vi "network stream read bulk.vi"(0 "endpoint in":refnum<k21>, 1 "Data num":i32, 3 "error in (no error)":errorcluster) -> (7 "endpoint out":refnum<k21>, 8 "Data":fxp<+/-,17,5>[](array[numeric]) format="%#_17g", 10 "error out":errorcluster)   [LabVIEW 2024]
uses:
  <resource>/objmgr/ni.dex.rc
panel:
  out "Data read num":i32
  out "Remaining data num":i32
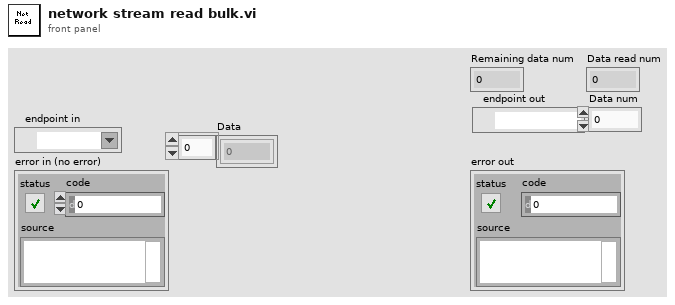
[diagram p1: front panel]
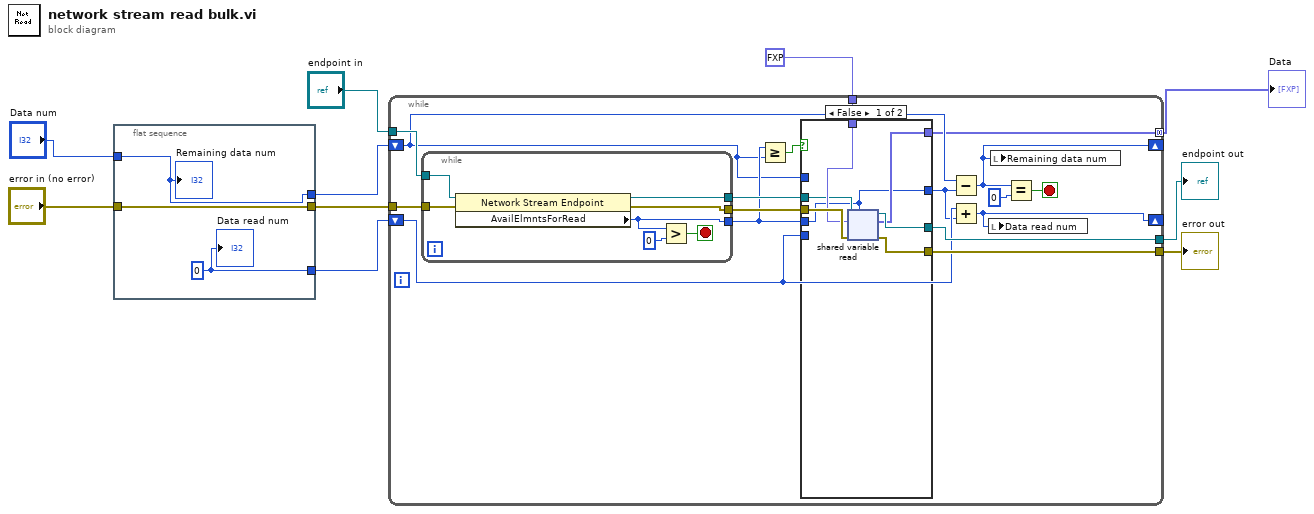
[diagram p0: block diagram]
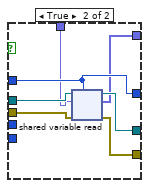
[diagram p2: hidden frame]
diagram:
  n1 = flat-sequence {
    tunnel: "error in (no error)" -> [w13]
    tunnel: [w13] -> w7
    tunnel: [w11] -> w5
    tunnel: [w12] -> w4
    tunnel: "Data num" -> [w11]
    frame #0 {
      w12 = 0 ("Data sent")
      "Remaining data num" <- w11
      "Data read num" <- w12
    }
  }
  n2 = while {
    tunnel: w7 -> [w29]
    tunnel: [w27] -> w9
    tunnel: "endpoint in" -> [w30]
    tunnel: [w26] -> w6
    shift-right: [w23] -> _
    shift-left: w5 -> [w17]
    shift-right: [w20] -> _
    shift-left: w4 -> [w22]
    tunnel: fxp<+/-,17,5> 0.0 ("Data 2") -> [w15]
    tunnel: [w14] -> w1 mode=concatenating
    stop <- w24 stop-if-true
    n3 = while {
      tunnel: w30 -> [w51]
      tunnel: w29 -> [w50]
      tunnel: [w47] -> w28
      tunnel: [w46] -> w18
      tunnel: [w45] -> w19
      stop <- w48 stop-if-true
      n4 = property class="Network Stream Endpoint"(reference=w51, error in=w50) -> (reference out=w45:refnum<k21>, error out=w47:errorcluster, "AvailElmntsForRead"=w46:i32)
      n5 = Greater?(x=w46, y=0) -> (0:w48:bool)
    }
    n6 = Greater Or Equal?(x=w18, y=w17) -> (x >= y?=w16:bool)
    n7 = case shown="False" w16 {
      tunnel: w19 -> [w34 w42]
      tunnel: w28 -> [w37 w44]
      tunnel: w22 -> [_ _]
      tunnel: w17 -> [_ w41]
      tunnel: [w36 w43] -> w27
      tunnel: [w33 w40] -> w26
      tunnel: [w31 w41] -> w21
      tunnel: w18 -> [w31 _]
      tunnel: w15 -> [w35 w39]
      tunnel: [w32 w38] -> w14
      frame False {
        n8 = shared-variable-read(w34, w37, w35, w31) -> (w33:refnum<k21>, w36:errorcluster, w32:fxp<+/-,17,5>[])  [unwired: 1 in, 1 out]
      }
      frame True {
        n9 = shared-variable-read(w42, w44, w39, w41) -> (w40:refnum<k21>, w43:errorcluster, w38:fxp<+/-,17,5>[])  [unwired: 1 in, 1 out]
      }
    }
    n10 = Subtract(x=w17, y=w21) -> (x-y=w23:i32)
    n11 = Add(x=w22, y=w21) -> (x+y=w20:i32)
    n12 = local write "Data read num"(w20) -> ()
    n13 = local write "Remaining data num"(w23) -> ()
    n14 = Equal?(x=w23, y=0) -> (x = y?=w24:bool)
  }
  "error out" <- w9
  "endpoint out" <- w6
  "Data" <- w1
